vi "Get Error Text.vi"(8 "error in":errorcluster, 10 "Language":u16(ring)=9 items=["Neutral"=0, "German"=7, "English"=9, "Spanish"=16, "French"=18, "Italian"=22], 11 "PCAN Error Code":u32) -> (0 "error out":errorcluster, 3 "PCAN Error Text":string)   [LabVIEW 2020, in "PCANBasic.lvlib"]
doc: "Returns a descriptive text of a given TPCANStatus error code, in any desired language.\nThe current languages available for translation are: \nNeutral (0x00), German (0x07), English (0x09), Spanish (0x0A),Italian (0x10) and French (0x0C)"
uses:
  PCANBasic.lvlib
  peak/PCANBasic64.dll
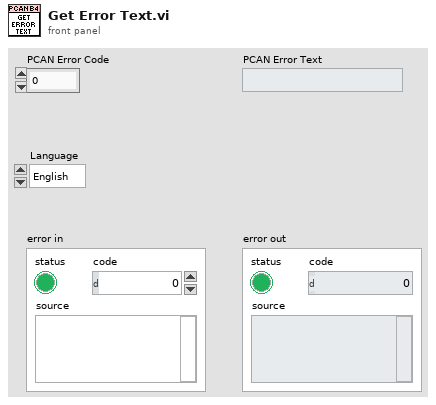
[diagram p1: front panel]
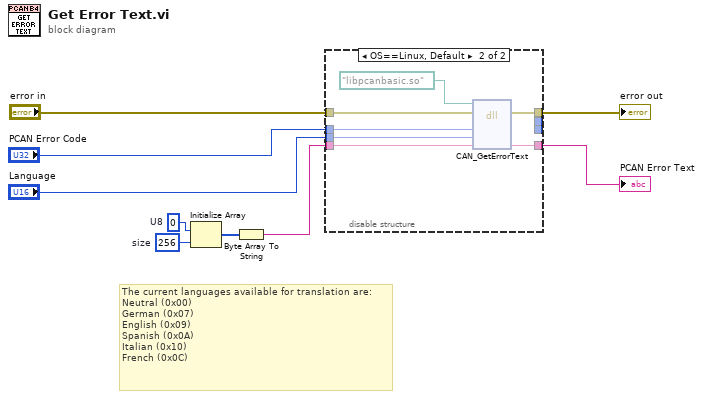
[diagram p0: block diagram]
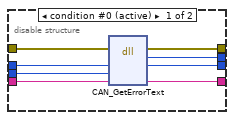
[diagram p2: hidden frame]
diagram:
  w5 = 256  # size
  w7 = u8 0  # U8
  # "The current languages available for translation are: \nNeutral (0x00)\nGerman (0x07)\nEnglish (0x09)\nSpanish (0x0A)\nItalian (0x10)\nFrench (0x0C)"
  n1 = Initialize Array(w7, w5) -> (w6:u8[])
  n2 = Byte Array To String(unsigned byte array=w6) -> (string=w4:string)
  n3 = disable-structure shown="OS==Linux, Default" {
    disable-tunnel: "Language" -> [w17 w24]
    disable-tunnel: w4 -> [w16 w23]
    disable-tunnel: [w15 w22] -> w3
    disable-tunnel: "PCAN Error Code" -> [w14 w21]
    disable-tunnel: "error in" -> [w13 w19]
    disable-tunnel: [w12 w18] -> w2
    disable-tunnel: [w11 _] -> _
    disable-tunnel: [w10 _] -> _
    frame condition #0 (active) {
      n4 = dll-call lib="D:/git/PCAN-Basic-LabVIEW/source/peak/PCANBasic*.dll" fn="CAN_GetErrorText" label="GetErrorText"(error in=w13, "Error"=w14, "Language"=w17, "Buffer"=w16) -> (error out=w12:errorcluster, "TPCANStatus"=w11:u32, "Error"=w10:u32, "Buffer"=w15:string)  [unwired: 3 in, 1 out]
    }
    frame condition #1 {
      n5 = dll-call lib="?" fn="CAN_GetErrorText" label="GetErrorText"(path in=path "libpcanbasic.so", error in=w19, "Error"=w21, "Language"=w24, "Buffer"=w23) -> (error out=w18:errorcluster, "Buffer"=w22:string)  [unwired: 4 in, 1 out]
    }
  }
  "error out" <- w2
  "PCAN Error Text" <- w3
